vi "FTW-URI-Build.vi"(0 "Base URI":string, 1 "Relative URI":string, 2 "Delimiter":string="/") -> (4 "Output":string)   [LabVIEW 2015]
uses:
  regex/FTW-Regex-Execute.vi
  error/FTW-ERR-ThrowGenericError.vi
  error/FTW-ERR-ThrowError.vi
  error/FTW-ERR-CallChain.vi
  error/FTW-ERR-NoErrorConstant.vi
  string/FTW-STR-ReplaceWhitespace.vi
  string/FTW-STR-Array-Delimit.vi
  regex/FTW-Regex-ReplaceAll.vi
  regex/FTW-Regex-Construct.vi
  lib/FTW-KernelFilepath.vi
  regex/FTW-Regex-Destroy.vi
panel:
  # "Inputs"
  # "Outputs"
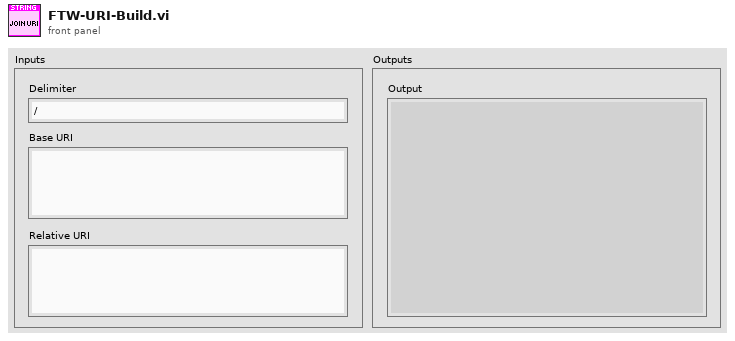
[diagram p1: front panel]
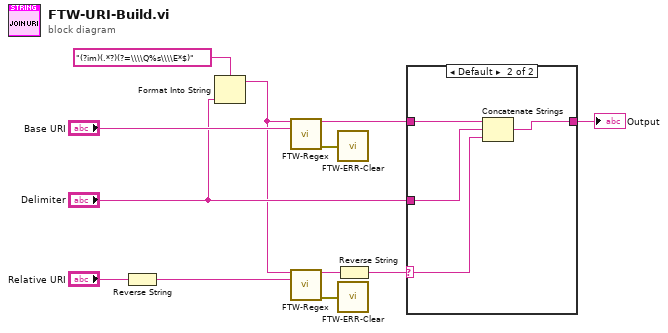
[diagram p0: block diagram]
diagram:
  n1 = Reverse String(1:"Relative URI") -> (0:w5:string)
  n2 = Format Into String(format string="(?im)(.*?)(?=\\\\Q%s\\\\E*$)" ("Regular Expression"), "Delimiter") -> (resulting string=w4:string)  [unwired: 2 in, 1 out]
  n3 = call "FTW-Regex.vi"("Regular Expression"=w4, "Input String"="Base URI") -> ("Match"=w10:string, "error out"=w3:errorcluster)  [unwired: 9 in, 3 out]
  n4 = call "FTW-Regex.vi"("Regular Expression"=w4, "Input String"=w5) -> ("Match"=w9:string, "error out"=w2:errorcluster)  [unwired: 9 in, 3 out]
  n5 = call "FTW-ERR-Clear.vi"("error to snuff"=w3) -> ()  [unwired: 1 out]
  n6 = call "FTW-ERR-Clear.vi"("error to snuff"=w2) -> ()  [unwired: 1 out]
  n7 = Reverse String(1:w9) -> (0:w1:string)
  n8 = case shown="Default" w1 {
    selector: w1 -> [_ w14]
    tunnel: w10 -> [w13 w17]
    tunnel: [w13 w16] -> w8
    tunnel: "Delimiter" -> [_ w15]
    frame "" {
    }
    frame Default {
      n9 = Concatenate Strings(w17, w15, w14) -> (w16:string)
    }
  }
  "Output" <- w8
